vi "创建-探头TCP连接.vi"(8 "超时(2s)":i32=2000, 11 "探头属性i":T1(array[cluster])) -> (0 "连接ID":refnum<k5>[](array[refnum]), 2 "连接数量":i32, 3 "探头属性o":T1(array[cluster]))   [LabVIEW 2016]
doc: "根据输入的属性中的 IP地址 与 端口 ，以Client身份创建 TCP连接，输出连接后的 探头属性 和 连接ID。"
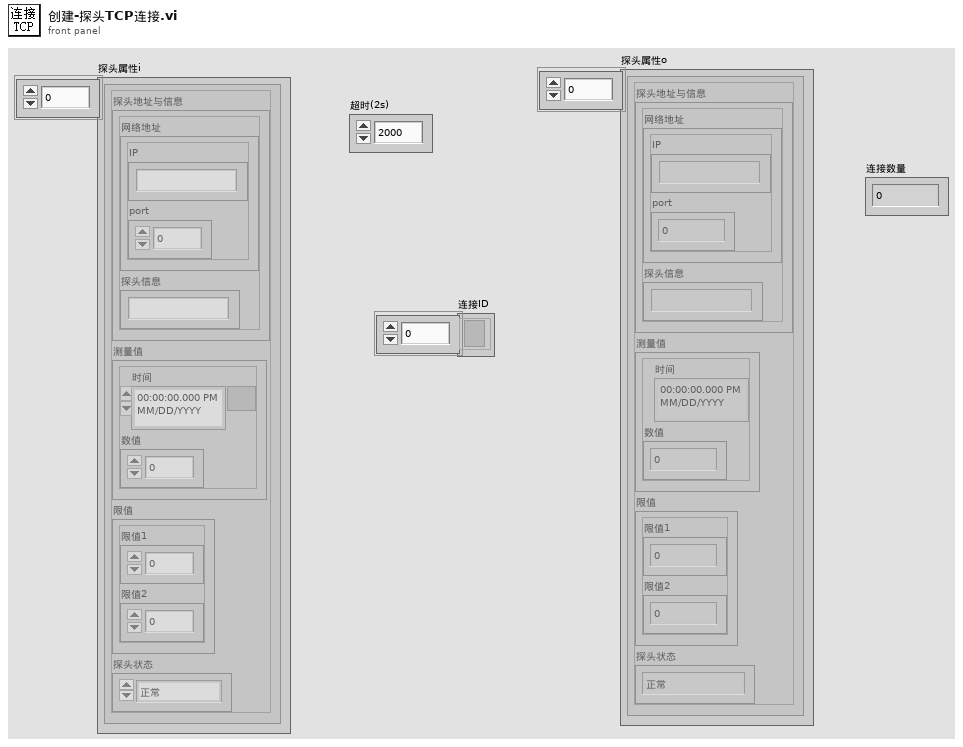
[diagram p1: front panel]
types:
  T1 = cluster{"探头地址与信息":cluster{"网络地址":cluster{"IP":string, "port":u16}, "探头信息":string}, "测量值":cluster{"时间":timestamp, "数值":dbl}, "限值":cluster{"限值1":dbl, "限值2":dbl}, "探头状态":enum16{"正常", "离线", "禁用", "一级报警", "二级报警"}}[]
  T2 = cluster{"探头地址与信息":cluster{"网络地址":cluster{"IP":string, "port":u16}, "探头信息":string}, "测量值":cluster{"时间":timestamp, "数值":dbl}, "限值":cluster{"限值1":dbl, "限值2":dbl}, "探头状态":enum16{"正常", "离线", "禁用", "一级报警", "二级报警"}}
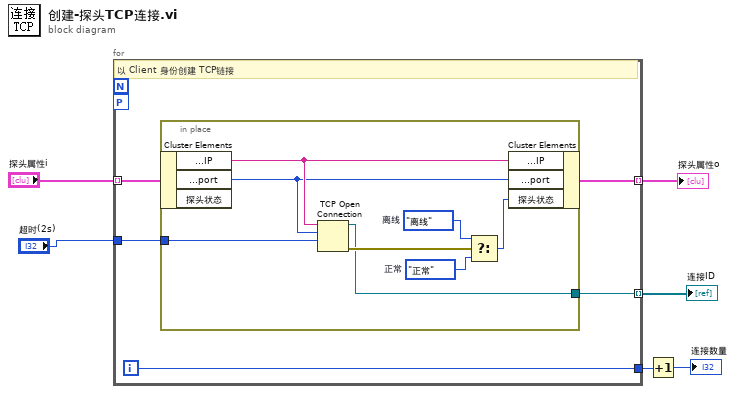
[diagram p0: block diagram]
diagram:
  n1 = for {
    tunnel: [w11] -> w4 mode=indexing
    tunnel: "探头属性i" -> [w10] mode=indexing
    workers-P: _ -> [_]
    tunnel: [w9] -> w5 mode=indexing
    tunnel: "超时(2s)" -> [w8]
    tunnel: [w7] -> w2
    i -> [w7]
    # "以 Client 身份创建 TCP链接"
    n2 = in-place {
      in-place-border: [w13] -> w11
      in-place-border: w8 -> [w12]
      w15 = enum16{"正常", "离线", "禁用", "一级报警", "二级报警"}."正常"  # 正常
      w16 = enum16{"正常", "离线", "禁用", "一级报警", "二级报警"}."离线"  # 离线
      n3 = in-place-cluster #1(w10) -> ("探头地址与信息.网络地址.IP"=w18:string, "探头地址与信息.网络地址.port"=w17:u16)  [unwired: 1 out]
      n4 = TCP Open Connection(address=w18, remote port or service name=w17, timeout ms (60000)=w12) -> (connection ID=w13:refnum<k5>, error out=w19:errorcluster)  [unwired: 2 in]
      n5 = Select(t=w16, s=w19, f=w15) -> (s? t:f=w14:enum16{"正常", "离线", "禁用", "一级报警", "二级报警"})
      n6 = in-place-cluster #1("探头地址与信息.网络地址.IP"=w18, "探头地址与信息.网络地址.port"=w17, "探头状态"=w14) -> (w9:T2)
    }
  }
  "探头属性o" <- w5
  "连接ID" <- w4
  n7 = Increment(x=w2) -> (x+1=→"连接数量":i32)
